vi "报表打印.vi"() -> ()   [LabVIEW 2014]
uses:
  <vilib>/printing/ReportDocExtensions.llb/Append Front Panel Image to Report (path).vi
  <vilib>/Utility/NIReport.llb/NI_report.lvclass
  <vilib>/Utility/NIReport.llb/NI_ReportGenerationCore.lvlib
  <vilib>/measure/NI_MABase.lvlib
panel:
  out "数组":dbl[](array[numeric])
  in  "number of copies (1)":i32=1 caption="打印份数"
  in  "?":bool
  in  "停止":bool
  in  "确定打印":bool
  in  "打印内容":enum16{"数组", "波形图", "前面板"}(ring)
  in  "amplitude":dbl=1.0 caption="幅值" format="%0.2p"
  in  "频率":dbl=5.0 format="%#_13g"
  in  "signal type":T1(ring) caption="信号类型"
  out "波形图":waveform(dbl)(graph)
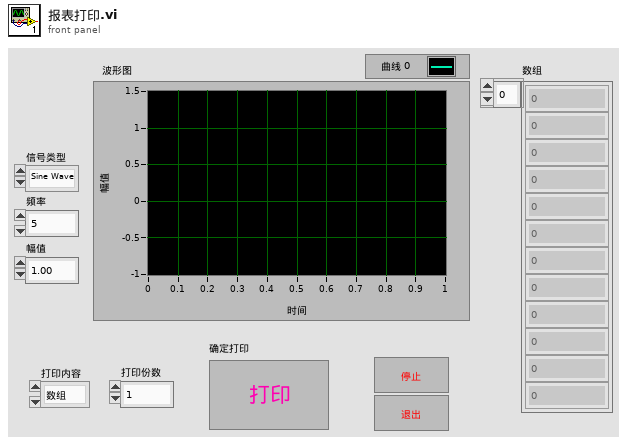
[diagram p1: front panel]
types:
  T1 = enum16{"Sine Wave", "Triangle Wave", "Square Wave", "Sawtooth Wave"}
  T2 = enum16{"Standard Report", "HTML", "Word", "Excel"}
  T3 = cluster{"top":dbl, "left":dbl, "right":dbl, "bottom":dbl}
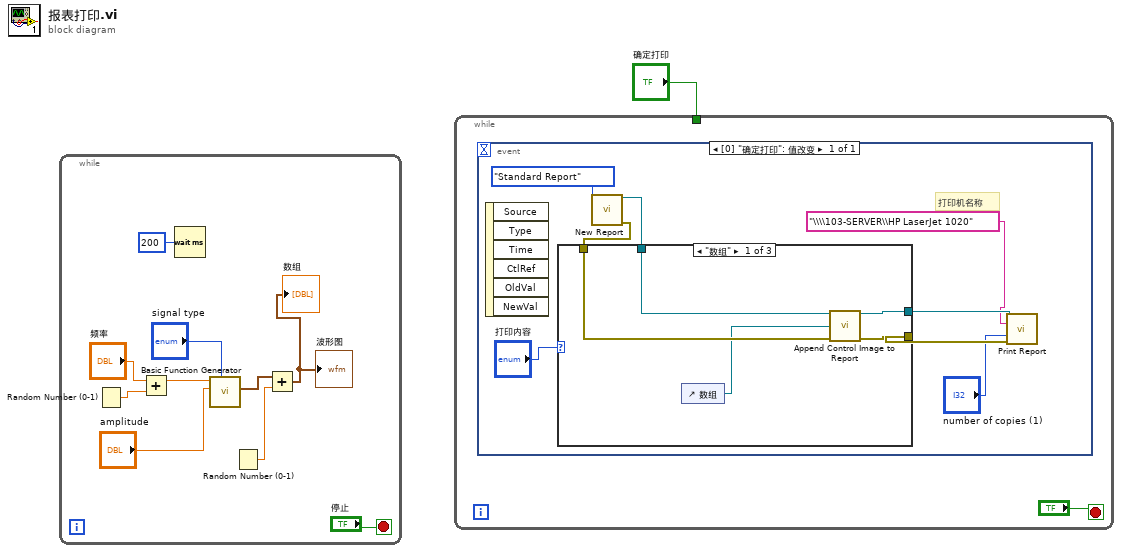
[diagram p0: block diagram]
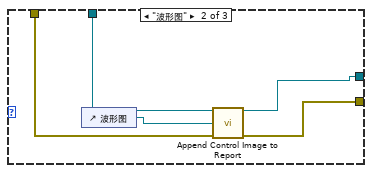
[diagram p2: hidden frame]
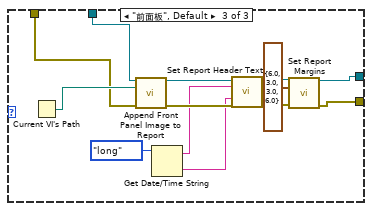
[diagram p3: hidden frame]
diagram:
  n1 = while {
    stop <- "停止" stop-if-true
    n2 = Random Number (0-1)() -> (number: 0 to 1=w4:dbl)
    n3 = Add(x="频率", y=w4) -> (x+y=w5:dbl)
    n4 = Wait (ms)(milliseconds to wait=u32 200 ("等待时间（毫秒）")) -> ()  [unwired: 1 out]
    n5 = call <vilib>:"Basic Function Generator.vi"("signal type"="signal type", "amplitude"="amplitude", "frequency"=w5) -> ("signal out"=w9:waveform(dbl))  [unwired: 6 in, 2 out]
    n6 = Random Number (0-1)() -> (number: 0 to 1=w8:dbl)
    n7 = Add(x=w9, y=w8) -> (x+y=→"波形图" →"数组":waveform(dbl))
  }
  n8 = while {
    tunnel: "确定打印" -> [_]
    stop <- "?" stop-if-true
    n9 = event shown="[0] \"确定打印\": 值改变" {
      selector: _ -> [_]
      dyn-events: _ -> [_]
      timeout: _ -> [_]
      event "确定打印": Value Change {
        # "打印机名称"
        n10 = event-data() -> ()  [unwired: 1 in, 6 out]
        n11 = call <vilib>:"New Report.vi"("report type"=T2."Standard Report") -> ("report out"=w17:refnum<class "NI_report.lvclass">, "error out"=w19:errorcluster)  [unwired: 13 in]
        n12 = case shown="\"数组\"" "打印内容" {
          tunnel: w17 -> [w22 w30 w31]
          tunnel: [w25 w28 w36] -> w16
          tunnel: [w24 w27 w37] -> w18
          tunnel: w19 -> [w23 w26 w42]
          frame "数组" {
            n13 = control-ref of="数组"() -> (w21:refnum<vi>)
            n14 = call-dynamic "Append Control Image to Report.vi"("report in"=w22, "ctrl reference"=w21, "error in (no error)"=w23) -> ("report out"=w25:refnum<class "NI_report.lvclass">, "error out"=w24:errorcluster)  [unwired: 9 in, 2 out]
          }
          frame "波形图" {
            n15 = control-ref of="波形图"() -> (w29:refnum<vi>)
            n16 = call-dynamic "Append Control Image to Report.vi"("report in"=w30, "ctrl reference"=w29, "error in (no error)"=w26) -> ("report out"=w28:refnum<class "NI_report.lvclass">, "error out"=w27:errorcluster)  [unwired: 9 in, 2 out]
          }
          frame "前面板", Default {
            n17 = Current VI's Path() -> (path=w43:path)
            n18 = call-poly <vilib>:"Append Front Panel Image to Report.vi"("report in"=w31, "VI"=w43, "error in (no error)"=w42) -> ("report out"=w41:refnum<class "NI_report.lvclass">, "error out"=w40:errorcluster)  [unwired: 8 in, 3 out]
            n19 = Get Date/Time String(date format (0)=enum16{"short", "long", "abbreviated"}."long" ("日期格式(0)")) -> (date string=w35:string, time string=w34:string)  [unwired: 2 in]
            n20 = call-dynamic "Set Report Header Text.vi"("report in"=w41, "left header text"=w35, "right header text"=w34, "error in (no error)"=w40) -> ("report out"=w39:refnum<class "NI_report.lvclass">, "error out"=w38:errorcluster)  [unwired: 10 in]
            n21 = call-dynamic "Set Report Margins.vi"("report in"=w39, "margins (1.00)"=T3 {"top"=6.0, "left"=3.0, "right"=3.0, "bottom"=6.0}, "error in (no error)"=w38) -> ("report out"=w36:refnum<class "NI_report.lvclass">, "error out"=w37:errorcluster)  [unwired: 10 in, 1 out]
          }
        }
        n22 = call-dynamic "Print Report.vi"("report in"=w16, "printer name (default)"="\\\\103-SERVER\\HP LaserJet 1020", "number of copies (1)"="number of copies (1)", "error in (no error)"=w18) -> ()  [unwired: 10 in, 2 out]
      }
    }
  }
